vi "_rsscope Get Value From Rng Table.vi"(8 "error in (no error)":errorcluster, 9 "Value":i32, 10 "Range Table Name":string, 11 "VISA resource name":refnum<visa-resource-name>) -> (0 "error out":errorcluster, 2 "Output Enum value":string, 3 "VISA resource name out":refnum<visa-resource-name>)   [LabVIEW 2014]
uses:
  rsidr_core.llb/rsscope_rsidr_core.lvlib
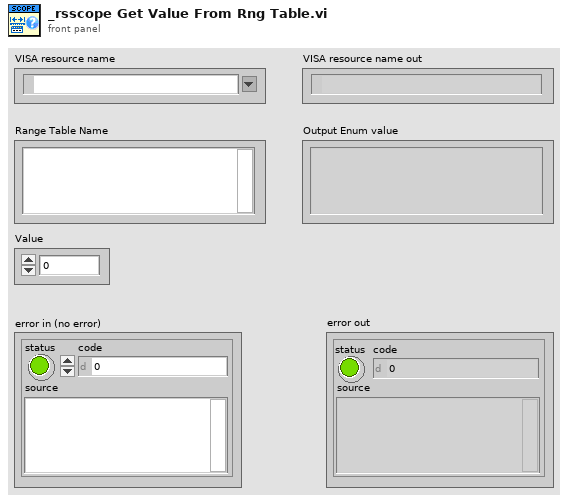
[diagram p1: front panel]
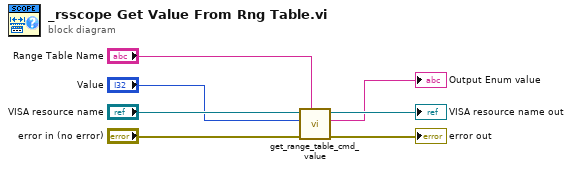
[diagram p0: block diagram]
diagram:
  n1 = call "get_range_table_cmd_value.vi"("Range Table ID in"="Range Table Name", "error in"="error in (no error)", "Input Int32 value"="Value", "VISA resource name"="VISA resource name") -> ("error out"=→"error out":errorcluster, "Cmd value out"=→"Output Enum value":string, "VISA resource name out"=→"VISA resource name out":refnum<visa-resource-name>)  [unwired: 5 in]
